vi "Drive_Utils_CalculateSpeed.vi"(6 "error in":errorcluster, 8 "Scaling factor":dbl=1.0, 9 "Speed current":dbl, 10 "delta Distance":dbl, 11 "Speed limit":dbl) -> (0 "error out":errorcluster, 3 "Speed":dbl)   [LabVIEW 2009, in "Drive.lvlib" / "Drive_Utils.lvlib"]
doc: "This VI calculates the speed based on current speed, distance to target point, current speed and scale factor. It used in position control algorithm.\n\nSpeed limit - max allowed speed. Should be positive.\ndelta Distance - distance to target. Could be positive or negative.\nSpeed current - current speed\nScaling factor - scales speed limit and drive constants. Use CalculateScale VI to get correct value."
uses:
  Drive_Utils.lvlib
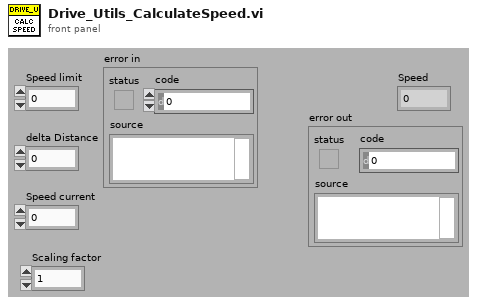
[diagram p1: front panel]
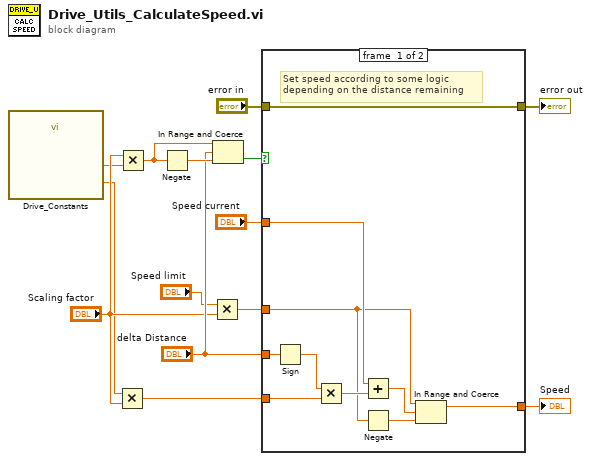
[diagram p0: block diagram]
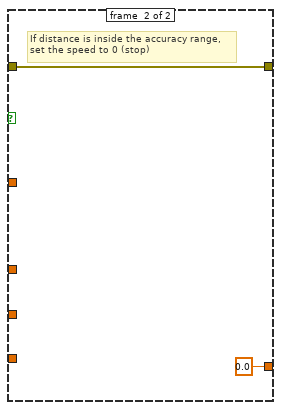
[diagram p2: hidden frame]
diagram:
  n1 = call "Drive_Constants.vi"() -> ("Position accuracy (m)"=w4:dbl, "Speed step (m/s)"=w3:dbl)  [unwired: 23 in, 3 out]
  n2 = Multiply(x=w3, y="Scaling factor") -> (x*y=w9:dbl)
  n3 = Multiply(x="Scaling factor", y=w4) -> (x*y=w8:dbl)
  n4 = Negate(x=w8) -> (-x=w13:dbl)
  n5 = Multiply(x="Speed limit", y="Scaling factor") -> (x*y=w7:dbl)
  n6 = In Range and Coerce(upper limit=w8, x="delta Distance", lower limit=w13) -> (In Range?=w14:bool)  [unwired: 1 out]
  n7 = case shown="False" w14 {
    tunnel: "Speed current" -> [w23 _]
    tunnel: w7 -> [w16 _]
    tunnel: [w18 0.0 ("Speed limit")] -> w11
    tunnel: "delta Distance" -> [w24 _]
    tunnel: w9 -> [w21 _]
    tunnel: "error in" -> [w15 w25]
    tunnel: [w15 w25] -> w1
    frame #0 {
      # "Set speed according to some logic\ndepending on the distance remaining"
      n8 = Sign(1:w24) -> (0:w22:dbl)
      n9 = Multiply(x=w22, y=w21) -> (x*y=w20:dbl)
      n10 = Add(x=w23, y=w20) -> (x+y=w19:dbl)
      n11 = Negate(x=w16) -> (-x=w17:dbl)
      n12 = In Range and Coerce(upper limit=w16, x=w19, lower limit=w17) -> (coerced(x)=w18:dbl)  [unwired: 1 out]
    }
    frame #1 {
      # "If distance is inside the accuracy range,\nset the speed to 0 (stop)"
    }
  }
  "Speed" <- w11
  "error out" <- w1
